vi "Comm_Send(SubVI).vi"(5 "High Priority?":bool, 7 "QueuSelector":T1, 8 "Error In":errorcluster, 10 "Data":variant, 11 "Command":T2=enum."WaitOnReport") -> (0 "error out":errorcluster)   [LabVIEW 2018, in "MainFrameLib.lvlib"]
uses:
  MainFrameLib.lvlib
  TypeDefs/Command_Enum.ctl
  TypeDefs/QNamesEnum.ctl
  TypeDefs/FGV_Enum.ctl
  TypeDefs/DataCluster.ctl
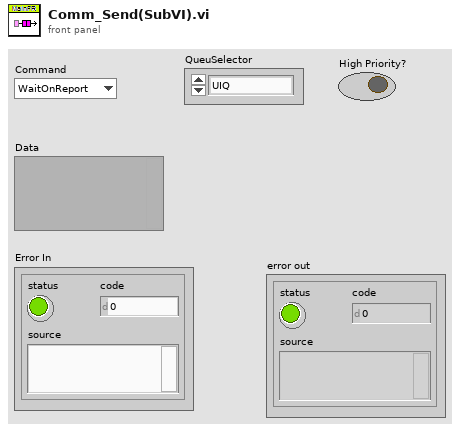
[diagram p1: front panel]
types:
  T1 = typedef "MainFrameLib.lvlib/QNamesEnum.ctl" = enum16{"UIQ", "ProcessQ", "CiscoQ", "KCSQ"}
  T2 = typedef "MainFrameLib.lvlib/Command_Enum.ctl" = enum16{"CheckSRLinks", "UpdateKCSColorCode", "StartLinkageCheck", "GetSRNotes", "DisplayAEStats", "InWork&Neglected", "RemapAENames", "ClearFolder", "UpdateReportsList", "ExcelReports", "TeamStats", "LoadReport", "WaitOnReport", "RequestReport", "Error", "Idle", "InitializeData", "ScreenPop", "Initialize", "UpdateCiscoAgentsView", "CancelRequests", "ClipboardCopy", "SaveNeglectedToFile", "Shutdown"}
  T3 = typedef "MainFrameLib.lvlib/DataCluster.ctl" = cluster{"Command":T2, "Data":variant}
  T4 = typedef "MainFrameLib.lvlib/FGV_Enum.ctl" = enum16{"Close", "GetRefs", "Initialize"}
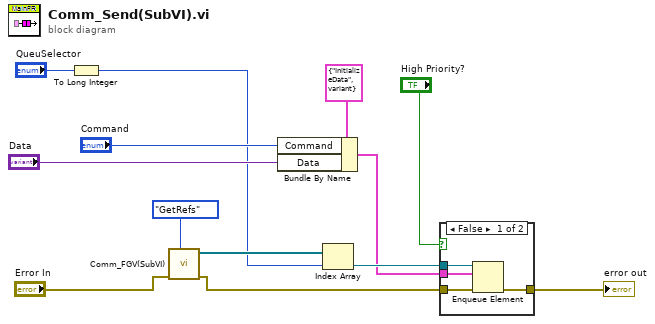
[diagram p0: block diagram]
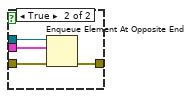
[diagram p2: hidden frame]
diagram:
  n1 = To Long Integer(number="QueuSelector") -> (32bit integer=w1:i32)
  n2 = call "Comm_FGV(SubVI).vi"("Enum"=FGV_Enum."GetRefs", "error in (no error)"="Error In") -> ("error out"=w9:errorcluster, "Array"=w13:refnum<queue>[])  [unwired: 8 in]
  n3 = Bundle By Name(cluster=T3 {"Command"=enum."InitializeData", "Data"=variant} ("element"), "Command"="Command", "Data"="Data") -> (w7:T3)
  n4 = Index Array(array=w13, index=w1) -> (element=w10:refnum<queue>)
  n5 = case shown="False" "High Priority?" {
    tunnel: w10 -> [w17 w19]
    tunnel: w9 -> [w16 w21]
    tunnel: w7 -> [w15 w18]
    tunnel: [w14 w20] -> w4
    frame False {
      n6 = Enqueue Element(queue=w17, element=w15, error in (no error)=w16) -> (error out=w14:errorcluster)  [unwired: 1 in, 2 out]
    }
    frame True {
      n7 = Enqueue Element At Opposite End(queue=w19, element=w18, error in (no error)=w21) -> (error out=w20:errorcluster)  [unwired: 1 in, 2 out]
    }
  }
  "error out" <- w4
